vi "_Unlock JKISMQ.vi"(8 "Error in":errorcluster caption="Error in (no error)", 11 "JKISMQ":T1) -> (0 "Error out":errorcluster, 3 "JKISMQ":T1)   [LabVIEW 2020, in "JKI-State-Machine-Plus.lvlib"]
uses:
  _JKISMQ.ctl
  _Cross JKI StateMachine State Data.ctl
  _Cross JKI StateMachine State Response.ctl
  JKI-State-Machine-Plus.lvlib
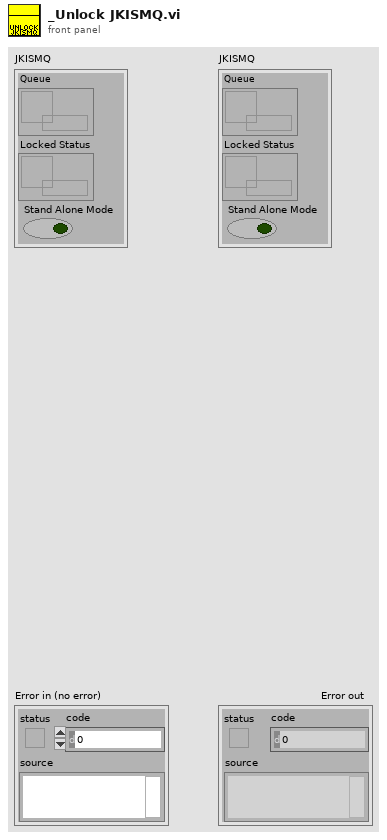
[diagram p1: front panel]
types:
  T1 = typedef "JKI-State-Machine-Plus.lvlib/_JKISMQ.ctl" = cluster{"Queue":refnum<queue>, "Locked Status":refnum<data-value>, "Stand Alone Mode":bool}
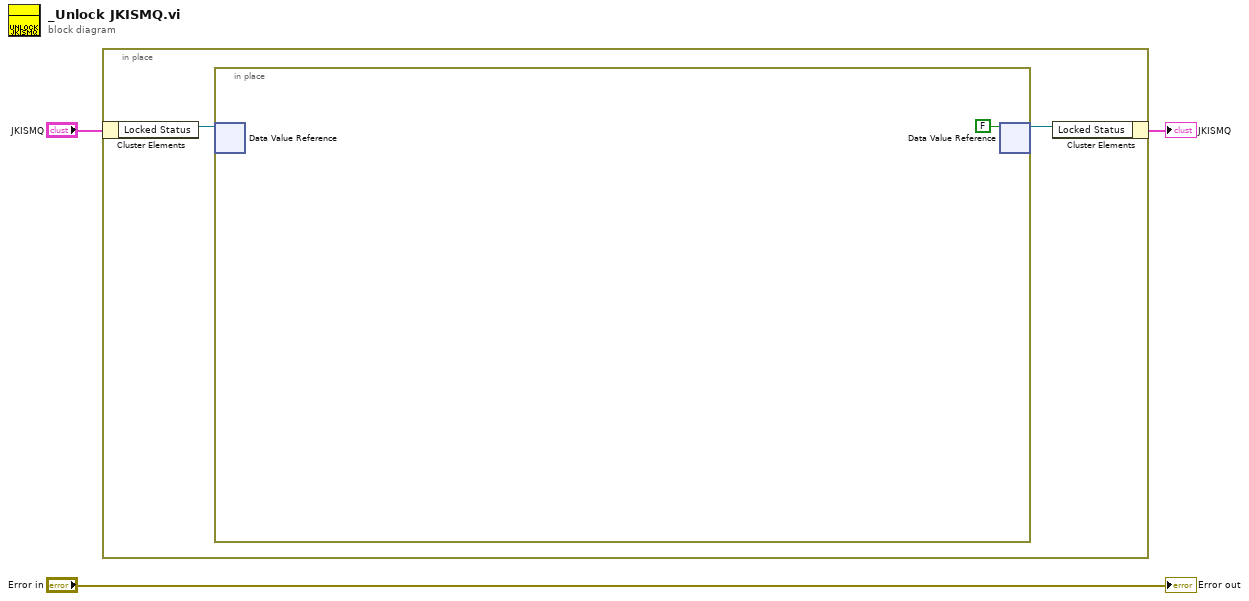
[diagram p0: block diagram]
diagram:
  n1 = in-place "In Place Element Structure" {
    n2 = in-place-cluster #1("JKISMQ") -> ("Locked Status"=w5:refnum<data-value>)
    n3 = in-place {
      n4 = in-place-dvr #2(w5) -> ()  [unwired: 2 out]
      n5 = in-place-dvr #2(FALSE ("data value")) -> (w4:refnum<data-value>)  [unwired: 1 out]
    }
    n6 = in-place-cluster #1("Locked Status"=w4) -> (→"JKISMQ":T1)
  }
  "Error out" <- "Error in"
